vi "Update Class Control.vi"(5 "LVClass":refnum<vi>, 8 "error in (no error)":errorcluster) -> (0 "error out":errorcluster)   [LabVIEW 2020, in "Conditum-Tools.lvlib" / "Entity Editor.lvclass"]
uses:
  Entity Editor.lvclass
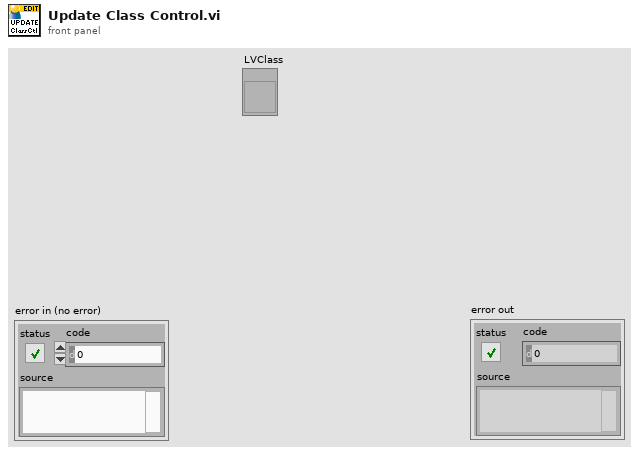
[diagram p1: front panel]
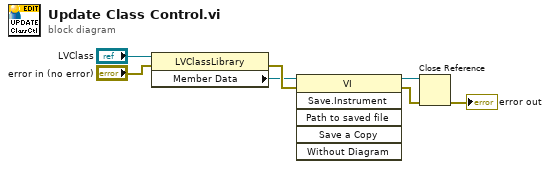
[diagram p0: block diagram]
diagram:
  n1 = property class="LVClassLibrary"(reference="LVClass", error in="error in (no error)") -> (error out=w7:errorcluster, "Member Data"=w4:refnum<vi>)  [unwired: 1 out]
  n2 = invoke class="VI" method="Save.Instrument"(reference=w4, error in=w7) -> (reference out=w5:refnum<vi>, error out=w6:errorcluster)  [unwired: 4 in, 4 out]
  n3 = Close Reference(reference=w5, error in (no error)=w6) -> (error out=→"error out":errorcluster)
